vi "Parse Geometric Element.vi"(8 "error in":errorcluster, 11 "Element In":refnum<class "Tree.lvclass">) -> (0 "error out":errorcluster, 2 "Geometric":refnum<class "Geometric.lvclass">[](array[class]), 3 "Element Out":refnum<class "Tree.lvclass">)   [LabVIEW 2019, in "ParseGDSII.lvclass"]
uses:
  ParseGDSII.lvclass
  Tree/Tree.lvclass
  DataTypes/Base/GDSII.DataType.lvclass
  Elements/Geometric.lvclass
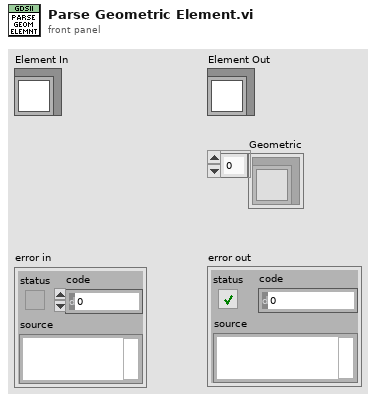
[diagram p1: front panel]
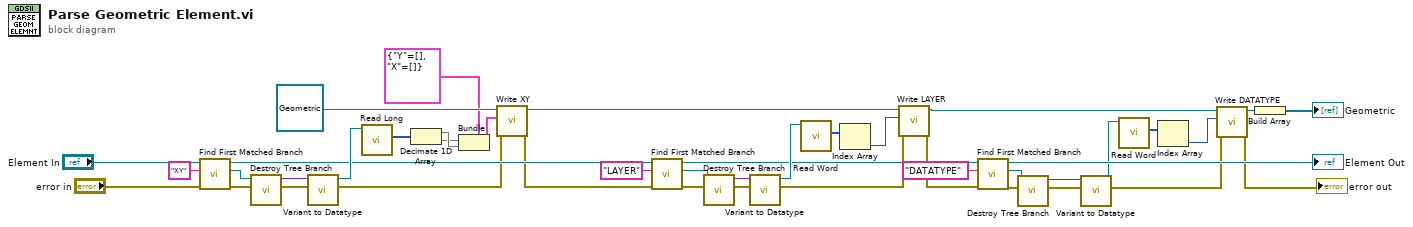
[diagram p0: block diagram]
diagram:
  n1 = call "Find First Matched Branch.vi"("error in"="error in", "Branch Name Exact"="XY", "Tree in"="Element In") -> ("error out"=w21:errorcluster, "Matched Branch"=w42:refnum<class "Tree.lvclass">, "Tree out"=w38:refnum<class "Tree.lvclass">)  [unwired: 5 in, 1 out]
  n2 = call "Destroy Tree Branch.vi"("error in"=w21, "Tree in"=w42) -> ("error out"=w28:errorcluster, "Root"=w41:variant)  [unwired: 8 in]
  n3 = call "Variant to Datatype.vi"("error in"=w28, "Variant"=w41) -> ("error out"=w20:errorcluster, "DataType"=w40:refnum<class "GDSII.DataType.lvclass">)  [unwired: 8 in]
  n4 = call-dynamic "Read Long.vi"("GDSII.DataType in"=w40) -> ("Long"=w39:i32[])  [unwired: 9 in, 1 out]
  n5 = Decimate 1D Array(w39) -> (w24:i32[], w23:i32[])
  n6 = Bundle(cluster=cluster{"Y":i32[], "X":i32[]} {"Y"=[], "X"=[]} ("XY"), "Y"=w23, "X"=w24) -> (w22:cluster{"Y":i32[], "X":i32[]})
  n7 = call-dynamic "Write XY.vi"("error in (no error)"=w20, "XY"=w22, "Element in"=refnum<class "Geometric.lvclass"> refnum ("Geometric")) -> ("error out"=w19:errorcluster, "Element out"=w12:refnum<class "Geometric.lvclass">)  [unwired: 7 in]
  n8 = call "Find First Matched Branch.vi"("error in"=w19, "Branch Name Exact"="LAYER", "Tree in"=w38) -> ("error out"=w16:errorcluster, "Matched Branch"=w35:refnum<class "Tree.lvclass">, "Tree out"=w31:refnum<class "Tree.lvclass">)  [unwired: 5 in, 1 out]
  n9 = call "Destroy Tree Branch.vi"("error in"=w16, "Tree in"=w35) -> ("error out"=w17:errorcluster, "Root"=w36:variant)  [unwired: 8 in]
  n10 = call "Variant to Datatype.vi"("error in"=w17, "Variant"=w36) -> ("error out"=w15:errorcluster, "DataType"=w34:refnum<class "GDSII.DataType.lvclass">)  [unwired: 8 in]
  n11 = call-dynamic "Read Word.vi"("GDSII.DataType in"=w34) -> ("Word"=w33:i16[])  [unwired: 9 in, 1 out]
  n12 = Index Array(array=w33) -> (element=w13:i16)  [unwired: 1 in]
  n13 = call-dynamic "Write LAYER.vi"("error in (no error)"=w15, "LAYER"=w13, "Geometric in"=w12) -> ("error out"=w14:errorcluster, "Geometric out"=w3:refnum<class "Geometric.lvclass">)  [unwired: 7 in]
  n14 = call "Find First Matched Branch.vi"("error in"=w14, "Branch Name Exact"="DATATYPE", "Tree in"=w31) -> ("error out"=w11:errorcluster, "Matched Branch"=w29:refnum<class "Tree.lvclass">, "Tree out"=→"Element Out":refnum<class "Tree.lvclass">)  [unwired: 5 in, 1 out]
  n15 = call "Destroy Tree Branch.vi"("error in"=w11, "Tree in"=w29) -> ("error out"=w10:errorcluster, "Root"=w30:variant)  [unwired: 8 in]
  n16 = call "Variant to Datatype.vi"("error in"=w10, "Variant"=w30) -> ("error out"=w6:errorcluster, "DataType"=w8:refnum<class "GDSII.DataType.lvclass">)  [unwired: 8 in]
  n17 = call-dynamic "Read Word.vi"("GDSII.DataType in"=w8) -> ("Word"=w7:i16[])  [unwired: 9 in, 1 out]
  n18 = Index Array(array=w7) -> (element=w4:i16)  [unwired: 1 in]
  n19 = call-dynamic "Write DATATYPE.vi"("error in (no error)"=w6, "DATATYPE"=w4, "Geometric in"=w3) -> ("error out"=→"error out":errorcluster, "Geometric out"=w2:refnum<class "Geometric.lvclass">)  [unwired: 7 in]
  n20 = Build Array(w2) -> (→"Geometric":refnum<class "Geometric.lvclass">[])
